vi "Create XLS.vi"(7 "sheetname":string="Sheet1", 8 "error in (no error)":errorcluster, 10 "File Name":path) -> (0 "error out":errorcluster)   [LabVIEW 2013]
uses:
  C:/PhaeronGit/LVNPOI/Resources/NPOI 2.1.1 dotnet2/NPOI.dll
  Resources/NPOI 2.1.1 dotnet2/NPOI.dll
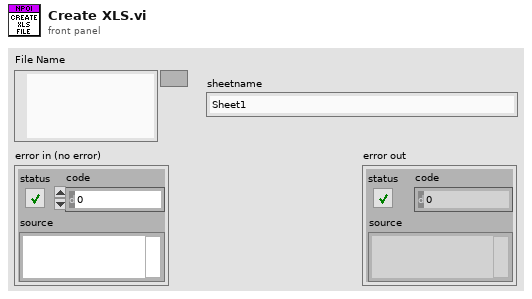
[diagram p1: front panel]
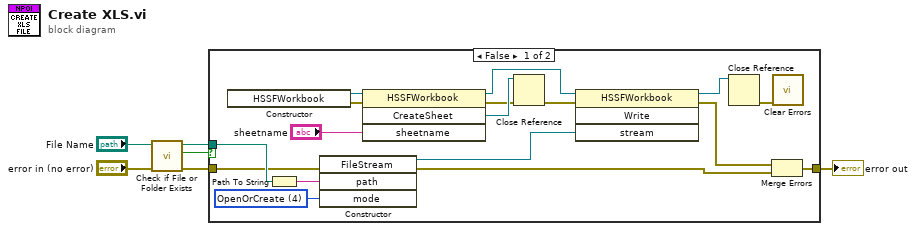
[diagram p0: block diagram]
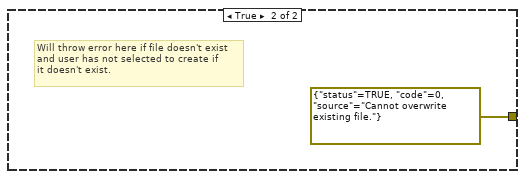
[diagram p2: hidden frame]
diagram:
  n1 = call <vilib>:"Check if File or Folder Exists.vi"("error in (no error)"="error in (no error)", "path"="File Name") -> ("error out"=w2:errorcluster, "file or folder exists?"=w1:bool, "dup path"=w3:path)  [unwired: 7 in]
  n2 = case shown="False" w1 {
    tunnel: [w17 errorcluster {"status"=TRUE, "code"=0, "source"="Cannot overwrite existing file."} ("error IO")] -> w6
    tunnel: w2 -> [w18 _]
    tunnel: w3 -> [w21 _]
    frame False {
      w23 = 4 items=["CreateNew"=1, "Create"=2, "Open"=3, "OpenOrCreate"=4, "Truncate"=5, "Append"=6] ("mode")
      n3 = constructor class="HSSFWorkbook"() -> (reference out=w11:refnum<k24>, error out=w10:errorcluster)  [unwired: 3 in, 1 out]
      n4 = Path To String(path=w21) -> (string=w22:string)
      n5 = constructor class="FileStream"(error in=w18, "path"=w22, "mode"=w23) -> (reference out=w20:refnum<k24>, error out=w15:errorcluster)  [unwired: 2 in, 3 out]
      n6 = invoke class="HSSFWorkbook" method="CreateSheet"(reference=w11, error in=w10, "sheetname"="sheetname") -> (reference out=w9:refnum<k24>, error out=w12:errorcluster, "CreateSheet"=w13:refnum<k24>)  [unwired: 1 in, 1 out]
      n7 = Close Reference(reference=w13, error in (no error)=w12) -> (error out=w8:errorcluster)
      n8 = invoke class="HSSFWorkbook" method="Write"(reference=w9, error in=w8, "stream"=w20) -> (reference out=w19:refnum<k24>, error out=w14:errorcluster)  [unwired: 1 in, 2 out]
      n9 = Close Reference(reference=w19) -> (error out=w16:errorcluster)  [unwired: 1 in]
      n10 = Merge Errors(w14, w15) -> (w17:errorcluster)
      n11 = call <vilib>:"Clear Errors.vi"("error in (no error)"=w16) -> ()  [unwired: 6 in, 1 out]
    }
    frame True {
      # "Will throw error here if file doesn't exist\nand user has not selected to create if\nit doesn't exist."
    }
  }
  "error out" <- w6
